vi "Teleop.vi"(10 "Match Info":T2={"Autonomous Elapsed Seconds"=0.0, "TeleOp Elapsed Seconds"=0.0, "Disabled Elapsed Seconds"=0.0, "Visited Autonomous"=FALSE, "Visited TeleOp"=FALSE, "Visited Disabled"=FALSE, "Autonomous Settings"={"Autonomous Style"=enum."Independent", "VI Refnum"=refnum}}, 11 "Call Context":T3) -> ()   [LabVIEW 2020]
doc: "This VI is called for each TeleOp packet received from the DS where the robot is not disabled. It is often used to read from the joysticks and update I/O or to update setpoints for timed control loops. It should complete and return within 20 milliseconds or it may miss DS packets."
uses:
  <vilib>/Rock Robotics/WPI/DriverStation/WPI_DriverStationDerivedRobotMode.ctl
  <vilib>/Rock Robotics/WPI/DriverStation/WPI_DriverStationMatch Info.ctl
  <vilib>/Rock Robotics/WPI/ThirdParty/Sensors/navX/_TypeDefs/FRIC_navX_DeviceNumbersTypeDef.ctl
  <vilib>/Rock Robotics/WPI/ThirdParty/REV Robotics/REVLib/Typedef/Spark MAX Control Type.ctl
  <vilib>/Rock Robotics/Network Tables/NT Write Number.vi
  <vilib>/Rock Robotics/Network Tables/NT Read Boolean.vi
  <vilib>/Rock Robotics/Network Tables/NT Read Number.vi
  <vilib>/Rock Robotics/WPI/Utilities/WPI_GetSetVariantRefNum.vi
panel:
  out "sensor Position":dbl
  out "select Teleop":i32
  out "Heading":dbl
  out "Pitch":dbl
  out "Roll":dbl
  out "Yaw":dbl
  out "Raw Values":T1 {"Accel X" format="%.8f"; "Accel Y" format="%.8f"; "Accel Z" format="%.8f"; "Gyro X" format="%.8f"; "Gyro Y" format="%.8f"; "Gyro Z" format="%.8f"; "Mag X" format="%.8f"; "Mag Y" format="%.8f"; "Mag Z" format="%.8f"}
  out "Gripper Command":dbl
  out "arm error out":errorcluster
  out "Sample Slider 0":dbl(slide) scale=0.0..5.0
  out "Sample Boolean 1":bool
  out "Sample Boolean 0":bool
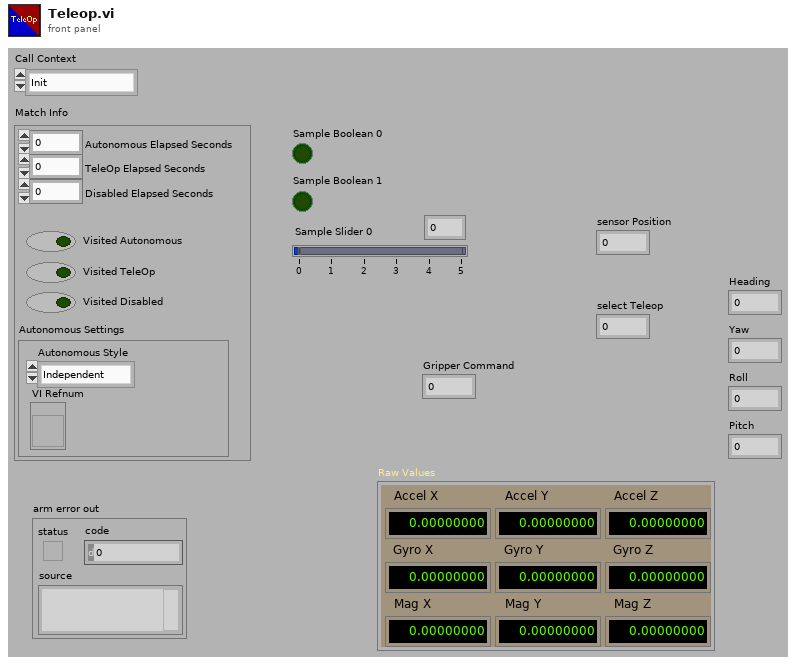
[diagram p1: front panel]
types:
  T1 = cluster{"Accel X":dbl, "Accel Y":dbl, "Accel Z":dbl, "Gyro X":dbl, "Gyro Y":dbl, "Gyro Z":dbl, "Mag X":dbl, "Mag Y":dbl, "Mag Z":dbl}
  T2 = typedef "WPI_DriverStationMatch Info.ctl" = cluster{"Autonomous Elapsed Seconds":dbl, "TeleOp Elapsed Seconds":dbl, "Disabled Elapsed Seconds":dbl, "Visited Autonomous":bool, "Visited TeleOp":bool, "Visited Disabled":bool, "Autonomous Settings":cluster{"Autonomous Style":enum16{"Iterative", "Independent"}, "VI Refnum":refnum<vi>}}
  T3 = typedef "WPI_DriverStationDerivedRobotMode.ctl" = enum16{"Init", "Execute", "Stop"}
  T4 = typedef "FRIC_navX_DeviceNumbersTypeDef.ctl" = enum16{"Dev0", "Dev1", "Dev2", "Dev3"}
  T5 = cluster{"Yaw":dbl, "Roll":dbl, "Pitch":dbl, "Heading":dbl, "Fused Heading":dbl}
  T6 = typedef "WPI_JoystickDevRef.ctl" = cluster{"Device":T7}
  T7 = typedef "WPI_JoystickDeviceEnum.ctl" = enum16{"USB 0", "USB 1", "USB 2", "USB 3", "USB 4", "USB 5"}
  T8 = typedef "WPI_MotorControlDeviceRef.ctl" = cluster{"DeviceStatus":errorcluster, "Type":T9, "PWM":cluster{"PWM Channel":T10, "DeadBand":T11}, "CAN":cluster{"Device Number":u8, "SetOutput VI Ref":variant, "GetOutput VI Ref":variant, "Enable VI Ref":variant, "Disable VI Ref":variant, "Data":variant}, "Invert":bool, "DIO PWM":cluster{"PWM \"Enable\" Channel":T10, "DIOChannel":T12, "PWM Rate":dbl}}
  T9 = typedef "WPI_MotorControlType.ctl" = enum16{"PWM", "CAN", "DIO PWM"}
  T10 = typedef "FPGA_DIOPWMChannel.ctl" = enum8{"PWM 0", "PWM 1", "PWM 2", "PWM 3", "PWM 4", "PWM 5", "PWM 6", "PWM 7", "PWM 8", "PWM 9", "PWM MXP 0", "PWM MXP 1", "PWM MXP 2", "PWM MXP 3", "PWM MXP 4", "PWM MXP 5", "PWM MXP 6", "PWM MXP 7", "PWM MXP 8", "PWM MXP 9", "Invalid"}
  T11 = typedef "WPI_PWMDeadband.ctl" = cluster{"Name":string, "maxPositivePwm":i32, "minPositivePwm":i32, "centerPwm":i32, "maxNegativePwm":i32, "minNegativePwm":i32, "angularRange":u16}
  T12 = typedef "FPGA_DIOChannel.ctl" = enum8{"DIO 0", "DIO 1", "DIO 2", "DIO 3", "DIO 4", "DIO 5", "DIO 6", "DIO 7", "DIO 8", "DIO 9", "DIO MXP 0", "DIO MXP 1", "DIO MXP 2", "DIO MXP 3", "DIO MXP 4", "DIO MXP 5", "DIO MXP 6", "DIO MXP 7", "DIO MXP 8", "DIO MXP 9", "DIO MXP 10", "DIO MXP 11", "DIO MXP 12", "DIO MXP 13", "DIO MXP 14", "DIO MXP 15", "SPI Port CS1", "SPI Port CS2", "SPI Port CS3", "SPI Port MISO", "SPI Port MOSI", "Invalid"}
  T13 = typedef "Spark MAX Control Type.ctl" = enum16{"Percent VBus", "Voltage", "Velocity", "Position", "Smart Motion", "Current", "Smart Velocity"}
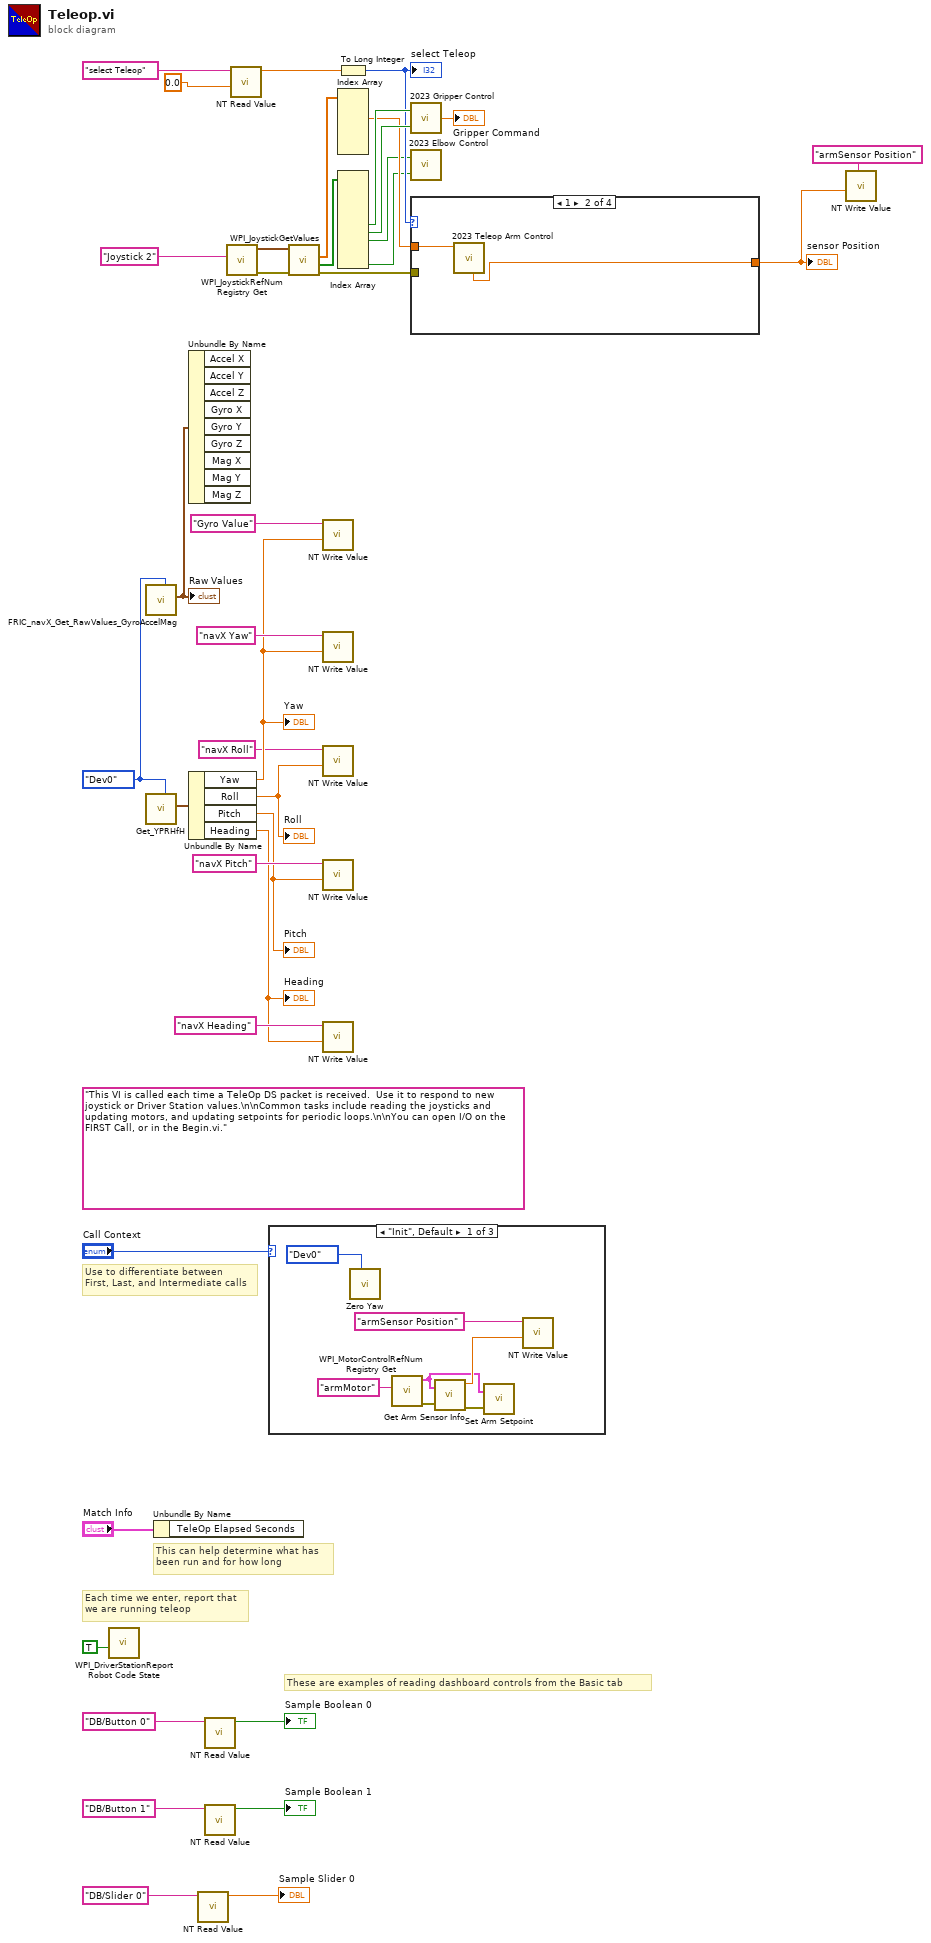
[diagram p0: block diagram]
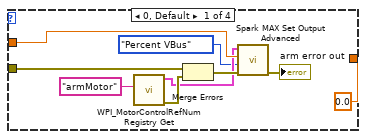
[diagram p4: hidden frame]
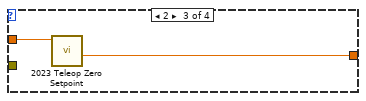
[diagram p5: hidden frame]
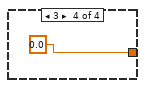
[diagram p6: hidden frame]
diagram:
  w22 = FRIC_navX_DeviceNumbersTypeDef."Dev0" ("Device Number")
  (unwired) "This VI is called each time a TeleOp DS packet is received.  Use it to respond to new joystick or Driver Station values.\n\nCommon tasks include reading the joysticks and updating motors, and updating setpoints for periodic loops.\n\nYou can open I/O on the FIRST Call, or in the Begin.vi."
  # "These are examples of reading dashboard controls from the Basic tab"
  # "Each time we enter, report that\nwe are running teleop"
  # "Use to differentiate between\nFirst, Last, and Intermediate calls"
  # "This can help determine what has\nbeen run and for how long"
  n1 = call <vilib>:"WPI_DriverStationReport Robot Code State.vi"("TeleOp"=TRUE ("Autonomous")) -> ()  [unwired: 10 in, 1 out]
  n2 = call <vilib>:"FRIC_navX_Get_RawValues_GyroAccelMag.vi"("Device Number"=w22) -> ("Raw Values (out)"=w23:T1)  [unwired: 10 in]
  "Raw Values" <- w23
  n3 = call <vilib>:"Get_YPRHfH.vi"("Device Number"=w22) -> ("YRPHfH"=w21:T5)  [unwired: 10 in]
  n4 = Unbundle By Name("Match Info") -> ()  [unwired: 1 out]
  n5 = Unbundle By Name(w23) -> ()  [unwired: 9 out]
  n6 = Unbundle By Name(w21) -> ("Yaw"=w18:dbl, "Roll"=w16:dbl, "Pitch"=w13:dbl, "Heading"=w12:dbl)
  "Yaw" <- w18
  "Roll" <- w16
  "Pitch" <- w13
  "Heading" <- w12
  n7 = call-poly <vilib>:"NT Read Value.vi"("name"="DB/Slider 0" ("refnum name")) -> ("value"=→"Sample Slider 0":dbl)  [unwired: 8 in, 2 out]
  n8 = call-poly <vilib>:"NT Read Value.vi"("name"="DB/Button 0" ("refnum name")) -> ("value"=→"Sample Boolean 0":bool)  [unwired: 8 in, 2 out]
  n9 = call-poly <vilib>:"NT Read Value.vi"("name"="DB/Button 1" ("refnum name")) -> ("value"=→"Sample Boolean 1":bool)  [unwired: 8 in, 2 out]
  n10 = call <vilib>:"WPI_JoystickRefNum Registry Get.vi"("refnum name"="Joystick 2") -> ("error out"=w30:errorcluster, "JoystickDevRef"=w29:T6)  [unwired: 1 in, 8 out]
  n11 = call-poly <vilib>:"NT Read Value.vi"("default value"=0.0, "name"="select Teleop") -> ("value"=w9:dbl)  [unwired: 7 in, 2 out]
  n12 = case shown="\"Init\", Default" "Call Context" {
    frame "Init", Default {
      n13 = call <vilib>:"Zero Yaw.vi"("Device Number"=FRIC_navX_DeviceNumbersTypeDef."Dev0") -> ()  [unwired: 11 in]
      n14 = call <vilib>:"WPI_MotorControlRefNum Registry Get.vi"("refnum name"="armMotor") -> ("error out"=w44:errorcluster, "MotorControlDevRef"=w41:T8)  [unwired: 9 in]
      n15 = call "Get Arm Sensor Info.vi"("MotorControlDevRef"=w41, "error in (no error)"=w44) -> ("Sensor Position"=w42:dbl, "error out"=w40:errorcluster)  [unwired: 2 out]
      n16 = call "Set Arm Setpoint.vi"("error in (no error)"=w40, "MotorControlDevRef in"=w41) -> ()  [unwired: 2 out]
      n17 = call-poly <vilib>:"NT Write Value.vi"("value"=w42, "name"="armSensor Position") -> ()  [unwired: 9 in, 1 out]
    }
    frame "Execute" {
    }
    frame "Stop" {
    }
  }
  n18 = call <vilib>:"WPI_JoystickGetValues.vi"("error in (no error)"=w30, "JoystickDevRef"=w29) -> ("error out"=w4:errorcluster, "Buttons"=w27:bool[], "Axes"=w31:dbl[])  [unwired: 5 in, 2 out]
  n19 = call-poly <vilib>:"NT Write Value.vi"("value"=w18, "name"="Gyro Value") -> ()  [unwired: 9 in, 1 out]
  n20 = call-poly <vilib>:"NT Write Value.vi"("value"=w18, "name"="navX Yaw") -> ()  [unwired: 9 in, 1 out]
  n21 = call-poly <vilib>:"NT Write Value.vi"("value"=w16, "name"="navX Roll") -> ()  [unwired: 9 in, 1 out]
  n22 = call-poly <vilib>:"NT Write Value.vi"("value"=w13, "name"="navX Pitch") -> ()  [unwired: 9 in, 1 out]
  n23 = call-poly <vilib>:"NT Write Value.vi"("value"=w12, "name"="navX Heading") -> ()  [unwired: 9 in, 1 out]
  n24 = To Long Integer(number=w9) -> (32bit integer=w8:i32)
  "select Teleop" <- w8
  n25 = Index Array(array=w31) -> (element #2=w5:dbl)  [unwired: 6 in, 5 out]
  n26 = Index Array(array=w27) -> (element #5=w25:bool, element #6=w26:bool, element #7=w3:bool, element #10=w2:bool)  [unwired: 10 in, 6 out]
  n27 = call "2023 Gripper Control.vi"("Button 6"=w26, "Button 5"=w25) -> ("Numeric"=→"Gripper Command":dbl)
  n28 = call "2023 Elbow Control.vi"("Button 6"=w2, "Button 5"=w3) -> ()  [unwired: 1 out]
  n29 = case shown="1" w8 {
    tunnel: [0.0 ("Sensor Position") w57 w58 0.0] -> w6
    tunnel: w5 -> [w53 w56 w59 _]
    tunnel: w4 -> [w51 _ _ _]
    frame 0, Default {
      n30 = call <vilib>:"WPI_MotorControlRefNum Registry Get.vi"("refnum name"="armMotor") -> ("error out"=w52:errorcluster, "MotorControlDevRef"=w48:T8)  [unwired: 9 in]
      n31 = Merge Errors(w51, w52) -> (w49:errorcluster)
      n32 = call <vilib>:"Spark MAX Set Output Advanced.vi"("error in (no error)"=w49, "Control Mode"=Spark_MAX_Control_Type."Percent VBus", "Setpoint"=w53, "MotorControlDevRef"=w48) -> ("error out"=→"arm error out":errorcluster)  [unwired: 6 in, 1 out]
    }
    frame 1 {
      n33 = call "2023 Teleop Arm Control.vi"("Joystick Y Axis"=w56) -> ("Sensor Position"=w57:dbl)  [unwired: 9 in, 1 out]
    }
    frame 2 {
      n34 = call "2023 Teleop Zero Setpoint.vi"("Joystick Y Axis"=w59) -> ("Commanded\nSet Output"=w58:dbl)  [unwired: 9 in, 1 out]
    }
    frame 3 {
    }
  }
  "sensor Position" <- w6
  n35 = call-poly <vilib>:"NT Write Value.vi"("value"=w6, "name"="armSensor Position") -> ()  [unwired: 9 in, 1 out]
